vi "Reporte_Excel.vi"() -> ()   [LabVIEW 2016]
uses:
  <vilib>/addons/_office/_exclsub.llb/font.ctl
  <vilib>/addons/_office/excel.llb/Excel Easy Table (num).vi
  <vilib>/Utility/NIReport.llb/Append Image to Report (path wrap).vi
  <vilib>/printing/ReportDocExtensions.llb/Append Front Panel Image to Report (path).vi
  <vilib>/printing/ReportDocExtensions.llb/Append VI Block Diagram to Report (path).vi
  <vilib>/Utility/NIReport.llb/NI_report.lvclass
  <vilib>/addons/_office/NI_ReportGenerationToolkit.lvlib
  <vilib>/Utility/NIReport.llb/NI_ReportGenerationCore.lvlib
panel:
  in  "Carpeta a Guardar":path=path "C:/Users/LuisFernando/Dropbox/6to Semestre/Instrumentacion Virtual/2017Mar23/Reporte.docx"
  in  "VI":path=path "C:/Users/LuisFernando/Dropbox/6to Semestre/Instrumentacion Virtual/2017Mar23/Reporte_Excel.vi"
  out "Gauge":dbl(knob) scale=0.0..10.0
  in  "path or URL of image":path=path "C:/Users/LuisFernando/Dropbox/6to Semestre/Instrumentacion Virtual/Masterchief.jpg"
  in  "Array":dbl[][](array[numeric])=[[1.0, 2.0, 3.0], [4.0, 5.0, 6.0], [7.0, 8.0, 9.0]]
  in  "String 2":string="Luis\nFernando\nZarazua\nAguilar"
  in  "String":string="Hola"
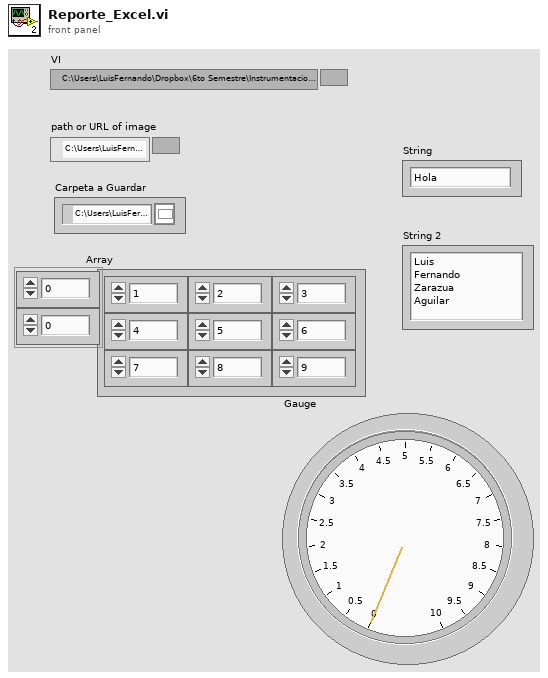
[diagram p1: front panel]
types:
  T1 = enum16{"xlColumnClustered", "xlColumnStacked", "xlColumnStacked100", "xl3DColumnClustered", "xl3DColumnStacked", "xl3DColumnStacked100", "xlBarClustered", "xlBarStacked", "xlBarStacked100", "xl3DBarClustered", "xl3DBarStacked", "xl3DBarStacked100", "xlLineStacked", "xlLineStacked100", "xlLineMarkers", "xlLineMarkersStacked", "xlLineMarkersStacked100", "xlPieOfPie", "xlPieExploded", "xl3DPieExploded", "xlBarOfPie", "xlXYScatterSmooth", "xlXYScatterSmoothNoMarkers", "xlXYScatterLines", "xlXYScatterLinesNoMarkers", "xlAreaStacked", "xlAreaStacked100", "xl3DAreaStacked", "xl3DAreaStacked100", "xlDoughnutExploded", "xlRadarMarkers", "xlRadarFilled", "xlSurface", "xlSurfaceWireframe", "xlSurfaceTopView", "xlSurfaceTopViewWireframe", "xlBubble", "xlBubble3DEffect", "xlStockHLC", "xlStockOHLC", "xlStockVHLC", "xlStockVOHLC", "xlCylinderColClustered", "xlCylinderColStacked", "xlCylinderColStacked100", "xlCylinderBarClustered", "xlCylinderBarStacked", "xlCylinderBarStacked100", "xlCylinderCol", "xlConeColClustered", "xlConeColStacked", "xlConeColStacked100", "xlConeBarClustered", "xlConeBarStacked", "xlConeBarStacked100", "xlConeCol", "xlPyramidColClustered", "xlPyramidColStacked", "xlPyramidColStacked100", "xlPyramidBarClustered", "xlPyramidBarStacked", "xlPyramidBarStacked100", "xlPyramidCol", "xl3DColumn", "xlLine", "xl3DLine", "xl3DPie", "xlPie", "xlXYScatter", "xl3DArea", "xlArea", "xlDoughnut", "xlRadar"}
  T2 = typedef "NI_ReportGenerationToolkit.lvlib/font.ctl" = cluster{"font name":string, "font size":dbl, "bold":u16, "italic":u16, "underline":u16, "strike through":u16, "font color":u32}
  T3 = enum16{"maximized", "minimized", "normal", "no change"}
  T4 = enum16{"Standard Report", "HTML", "Word", "Excel"}
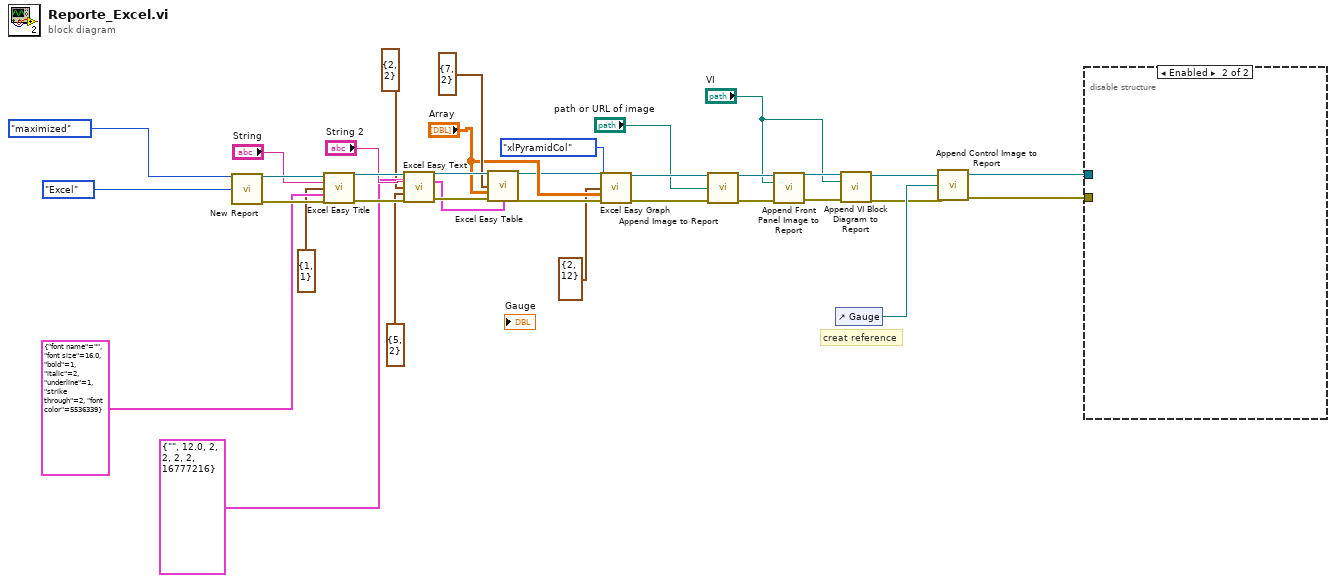
[diagram p0: block diagram]
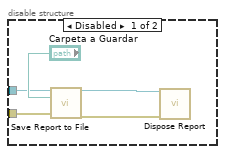
[diagram p2: hidden frame]
diagram:
  # "creat reference"
  n1 = call <vilib>:"New Report.vi"("window state (normal)"=T3."maximized", "report type"=T4."Excel") -> ("report out"=w33:refnum<class "NI_report.lvclass">, "error out"=w29:errorcluster)  [unwired: 12 in]
  n2 = call <vilib>:"Excel Easy Title.vi"("report in"=w33, "title"="String", "start (0, 0)"=cluster{"row":i32, "column":i32} {"row"=1, "column"=1}, "font"=T2 {"font name"="", "font size"=16.0, "bold"=1, "italic"=2, "underline"=1, "strike through"=2, "font color"=5536339}, "error in (no error)"=w29) -> ("report out"=w31:refnum<class "NI_report.lvclass">, "error out"=w28:errorcluster)  [unwired: 8 in, 1 out]
  n3 = call <vilib>:"Excel Easy Text.vi"("report in"=w31, "font"=T2 {"font name"="", "font size"=12.0, "bold"=2, "italic"=2, "underline"=2, "strike through"=2, "font color"=16777216}, "text"="String 2", "start (-1, -1)"=cluster{"row":i32, "column":i32} {"row"=2, "column"=2}, "end (-1, -1)"=cluster{"row":i32, "column":i32} {"row"=5, "column"=2}, "error in (no error)"=w28) -> ("report out"=w27:refnum<class "NI_report.lvclass">, "font out"=w23:T2, "error out"=w26:errorcluster)  [unwired: 5 in, 2 out]
  n4 = call-poly <vilib>:"Excel Easy Table.vi"("report in"=w27, "font"=w23, "start (0, 0)"=cluster{"row":i32, "column":i32} {"row"=7, "column"=2}, "text data"="Array", "error in (no error)"=w26) -> ("report out"=w1:refnum<class "NI_report.lvclass">, "error out"=w21:errorcluster)  [unwired: 6 in, 3 out]
  n5 = call <vilib>:"Excel Easy Graph.vi"("report in"=w1, "graph type (col clustered)"=T1."xlPyramidCol", "start (0, 0)"=cluster{"row":i32, "column":i32} {"row"=2, "column"=12}, "data"="Array", "error in (no error)"=w21) -> ("report out"=w20:refnum<class "NI_report.lvclass">, "error out"=w19:errorcluster)  [unwired: 9 in]
  n6 = call-poly <vilib>:"Append Image to Report.vi"("report in"=w20, "path or URL of image"="path or URL of image", "error in (no error)"=w19) -> ("report out"=w14:refnum<class "NI_report.lvclass">, "error out"=w13:errorcluster)  [unwired: 9 in, 2 out]
  n7 = call-poly <vilib>:"Append Front Panel Image to Report.vi"("report in"=w14, "VI"="VI", "error in (no error)"=w13) -> ("report out"=w16:refnum<class "NI_report.lvclass">, "error out"=w15:errorcluster)  [unwired: 8 in, 3 out]
  n8 = control-ref of="Gauge"() -> (w17:refnum<vi>)
  n9 = call-poly <vilib>:"Append VI Block Diagram to Report.vi"("report in"=w16, "VI"="VI", "error in (no error)"=w15) -> ("report out"=w11:refnum<class "NI_report.lvclass">, "error out"=w10:errorcluster)  [unwired: 8 in, 3 out]
  n10 = call-dynamic "Append Control Image to Report.vi"("report in"=w11, "ctrl reference"=w17, "error in (no error)"=w10) -> ("report out"=w9:refnum<class "NI_report.lvclass">, "error out"=w8:errorcluster)  [unwired: 9 in, 2 out]
  n11 = disable-structure shown="Enabled" {
    disable-tunnel: w9 -> [w37 _]
    disable-tunnel: w8 -> [w36 _]
    frame Disabled {
      n12 = call-dynamic "Save Report to File.vi"("report in"=w37, "report file path"="Carpeta a Guardar", "error in (no error)"=w36) -> ("report out"=w39:refnum<class "NI_report.lvclass">, "error out"=w38:errorcluster)  [unwired: 11 in]
      n13 = call-dynamic "Dispose Report.vi"("report in"=w39, "error in (no error)"=w38) -> ()  [unwired: 13 in, 1 out]
    }
    frame Enabled {
    }
  }
